vi "VII Read Bytes.vi"(5 "Len":u16, 6 "SubAddr":i32, 7 "SlaveAddr":u16, 9 "I2CIndex":i32, 10 "DevIndex":i32, 11 "DevType":i32) -> (2 "function return":i32, 3 "pReadData":u8[](array[numeric]))   [LabVIEW 2010, in "ControlI2C.lvlib"]
doc: "int __stdcall VII_ReadBytes(int DevType,int DevIndex,int I2CIndex,unsigned short SlaveAddr,int SubAddr,unsigned char *pReadData,unsigned short Len);"
uses:
  ControlI2C.lvlib
  ControlI2C/Ginkgo_Driver.dll
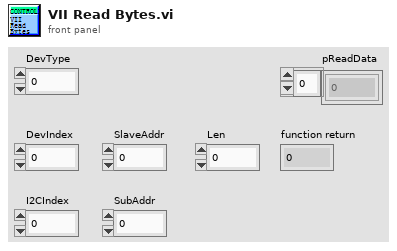
[diagram p1: front panel]
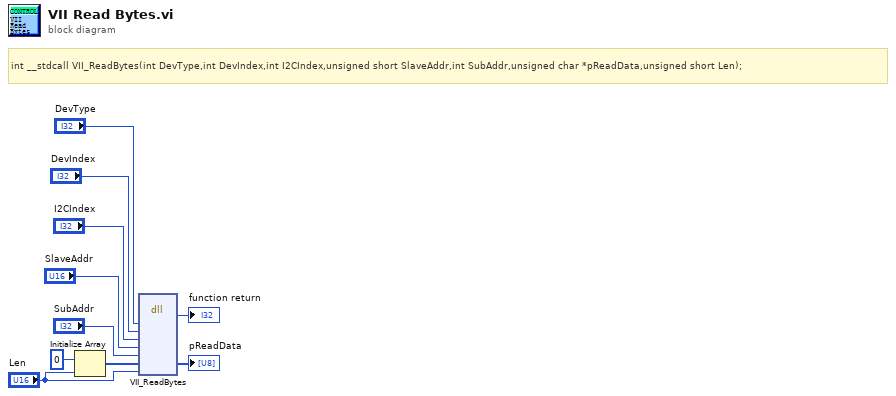
[diagram p0: block diagram]
diagram:
  # "int __stdcall VII_ReadBytes(int DevType,int DevIndex,int I2CIndex,unsigned short SlaveAddr,int SubAddr,unsigned char *pReadData,unsigned short Len);"
  n1 = Initialize Array(u8 0 ("element"), "Len") -> (w4:u8[])
  n2 = dll-call lib="E:/Project/vt_ginkgo/truck/Ginkgo Driver/vs2010/Ginkgo_USB-I2C&SPI&CAN_API_v2.0.3.3/lib/labview_32bit/ControlI2C/Ginkgo_Driver.*" fn="VII_ReadBytes"("DevType"="DevType", "DevIndex"="DevIndex", "I2CIndex"="I2CIndex", "SlaveAddr"="SlaveAddr", "SubAddr"="SubAddr", "pReadData"=w4, "Len"="Len") -> (→"function return":i32, "pReadData"=→"pReadData":u8[])  [unwired: 9 in, 2 out]
